vi "To Generic.vi"(8 "error in (no error)":errorcluster, 11 "Request Data in":refnum<class "Request Data.lvclass">) -> (0 "error out":errorcluster, 2 "Generic Data":refnum<class "Generic Data.lvclass">[](array[class]), 3 "Data Name":string[](array[string]))   [LabVIEW 2020, in "Publisher.lvlib" / "Request Data.lvclass"]
doc: "Present private data as an array of named generic data elements."
uses:
  Request Data.lvclass
  PPL/HDH.Data.Generic.lvlibp/Generic Data/Generic Data.lvclass
  Request Data.lvclass/Request Data.ctl
  PPL/HDH.Data.Generic.lvlibp/Data.lvclass
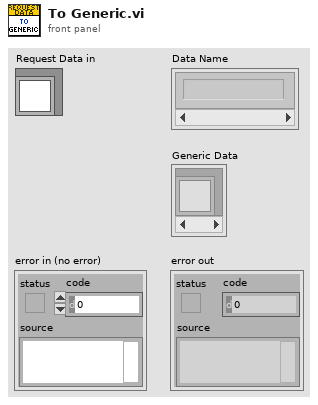
[diagram p1: front panel]
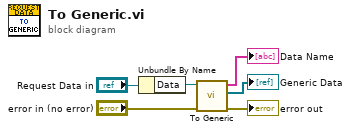
[diagram p0: block diagram]
diagram:
  n1 = Unbundle By Name("Request Data in") -> ("Data"=w5:refnum<class "Data.lvclass">)
  n2 = call-dynamic "To Generic.vi"("error in (no error)"="error in (no error)", "Data in"=w5) -> ("error out"=→"error out":errorcluster, "Generic Data"=→"Generic Data":refnum<class "Generic Data.lvclass">[], "Data Name"=→"Data Name":string[])  [unwired: 7 in]
